vi "error_check_Lakeshore336.vi"(8 "error in (no error)":errorcluster, 11 "VISA Refnum in":refnum<visa-resource-name>) -> (0 "error out":errorcluster, 3 "Session Out":refnum<visa-resource-name>)   [LabVIEW 2016]
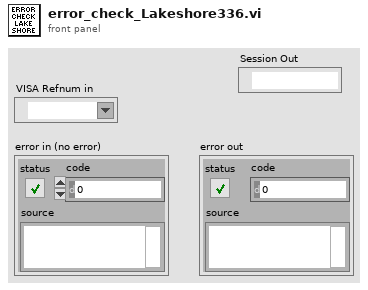
[diagram p1: front panel]
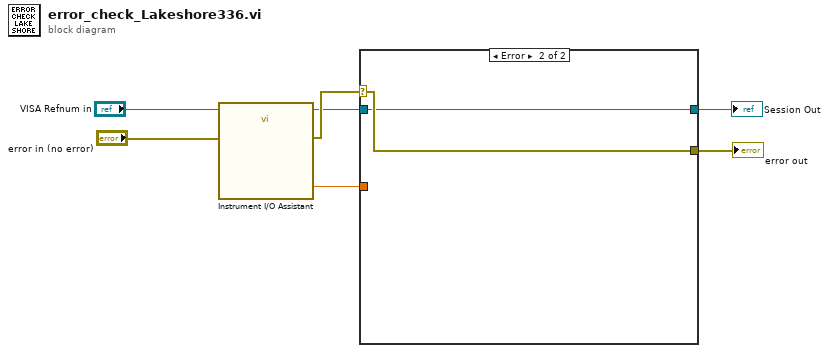
[diagram p0: block diagram]
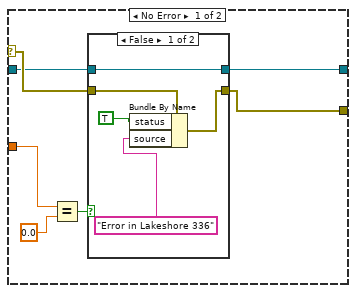
[diagram p2: hidden frame]
diagram:
  n1 = call "Instrument I/O Assistant"("Session In"="VISA Refnum in", "error in"="error in (no error)") -> ("Session Out"=w2:refnum<visa-resource-name>, "test_result"=w6:dbl, "error out"=w3:errorcluster)  [unwired: 23 in]
  n2 = case shown="Error" w3 {
    selector: w3 -> [w11 w23]
    tunnel: [w10 w23] -> w7
    tunnel: w6 -> [w12 _]
    tunnel: w2 -> [w9 w22]
    tunnel: [w8 w22] -> w1
    frame No Error {
      n3 = Equal?(x=w12, y=0.0) -> (x = y?=w14:bool)
      n4 = case shown="False" w14 {
        tunnel: w11 -> [w19 w21]
        tunnel: [w17 w21] -> w10
        tunnel: w9 -> [w16 w20]
        tunnel: [w16 w20] -> w8
        frame False {
          n5 = Bundle By Name(cluster=w19, "status"=TRUE, "source"="Error in Lakeshore 336") -> (w17:errorcluster)
        }
        frame True {
        }
      }
    }
    frame Error {
    }
  }
  "error out" <- w7
  "Session Out" <- w1
